vi "Msg Action.vi"(0 "TCP Server in":refnum<class "TCP Server.lvclass">, 1 "TCP Client ID":refnum<k5>, 2 "Sender IP":string, 5 "TCP Server Msg Actions":T1, 7 "uService ID":string, 9 "uService Class Name":string, 11 "error in (no error)":errorcluster) -> (4 "TCP Server out":refnum<class "TCP Server.lvclass">, 6 "External Error out":errorcluster, 15 "error out":errorcluster)   [LabVIEW 2026, in "TALOS.lvlib" / "TCP Server.lvlib" / "TCP Server.lvclass"]
uses:
  TCP Server.lvclass
  TCP Server Msg Actions.ctl
  C:/LabVIEW Code/TALOS/builds/Actor Framework PPL/Actor Framework.lvlibp/1abvi3w/vi.lib/ActorFramework/Actor/Actor.lvclass
  C:/LabVIEW Code/TALOS/talos/Father of all uServices/Father of all uServices/Father of all uServices.lvclass
  Ancestor/Ancestor/Ancestor.lvclass/Ancestor.ctl
  Guardian/Guardian Messages/Launch uService Msg/Launch uService Msg.lvclass/Launch uService Msg.ctl
  Guardian/Guardian Messages/Message to uService Msg/Message to uService Msg.lvclass/Message to uService Msg.ctl
  Guardian/Guardian Messages/TCP-SV Message Interpreter Msg/TCP-SV Message Interpreter Msg.lvclass/TCP-SV Message Interpreter Msg.ctl
  <vilib>/AdvancedString/Delimited String to 1D String Array (string).vi
  <vilib>/Utility/error.llb/Trim Whitespace (string).vi
  FGV/Error Memory/Get Error Description.vi
  Ancestor/Ancestor/Read ID.vi
  Support VIs/Get Class Name.vi
  Guardian/Guardian Messages/Message to uService Msg/Send Message to uService.vi
  <vilib>/Utility/error.llb/Trim Whitespace One-Sided.vi
  FGV/Error Memory/Error Memory Core.vi
  Support VIs/Circus Root Path.vi
  FGV/Error Memory/Error Crt Lvl checker.vi
  FGV/Error Memory/Error Memory Core.vi/40c8088d-b597-4017-91af-faa98e00292e.vi
  FGV/Error Memory/Error Memory Core.vi/d4a3ab98-063c-4e44-b43d-fbdcfe6c2be2.vi
  Father of all uServices/Father of all uServices/Father of all uServices.lvclass
  Support VIs/Global Memory.vi
  <vilib>/Utility/LVClass/Get LV Class Name.vi
  Support VIs/Is in Packed Library.vi
  Support VIs/TALOS Root path.vi
  Support VIs/Read CSV worksheet.vi
  Support VIs/Global Constants.vi
  <vilib>/Utility/error.llb/General Error Handler.vi
  Support VIs/Error Log.vi
  <vilib>/Utility/config.llb/Open Config Data.vi
  <vilib>/Utility/config.llb/Get Section Names.vi
  <vilib>/Utility/config.llb/Get Key Names.vi
  <vilib>/Utility/config.llb/Read Key.vi
  <vilib>/Utility/config.llb/Read Key (String).vi
  <vilib>/Utility/config.llb/Close Config Data.vi
  builds/Actor Framework PPL/Actor Framework.lvlibp/1abvi3w/vi.lib/ActorFramework/Message Enqueuer/Enqueue.vi
  Ancestor/Ancestor/Ancestor.lvclass
  <vilib>/Comparison/Equal/Equal Functor/Equal Functor.lvclass
  Guardian/Guardian Messages/Launch uService Msg/Launch uService Msg.lvclass
  Guardian/Guardian Messages/Message to uService Msg/Message to uService Msg.lvclass
  Guardian/Guardian Messages/TCP-SV Message Interpreter Msg/TCP-SV Message Interpreter Msg.lvclass
  builds/Actor Framework PPL/Actor Framework.lvlibp/1abvi3w/vi.lib/ActorFramework/Actor/Actor.lvclass
  TALOS.lvlib
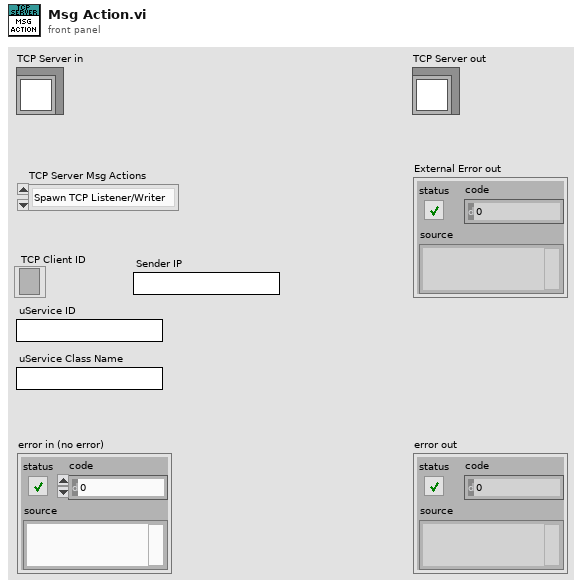
[diagram p1: front panel]
types:
  T1 = typedef "TALOS.lvlib/TCP Server.lvlib/TCP Server.lvclass/TCP Server Msg Actions.ctl" = enum16{"Spawn TCP Listener/Writer", "External Error", "I Exist", "Who the hell is this guy?", "Do nothing", "Are you the Bearer", "Farewell", "External Message"}
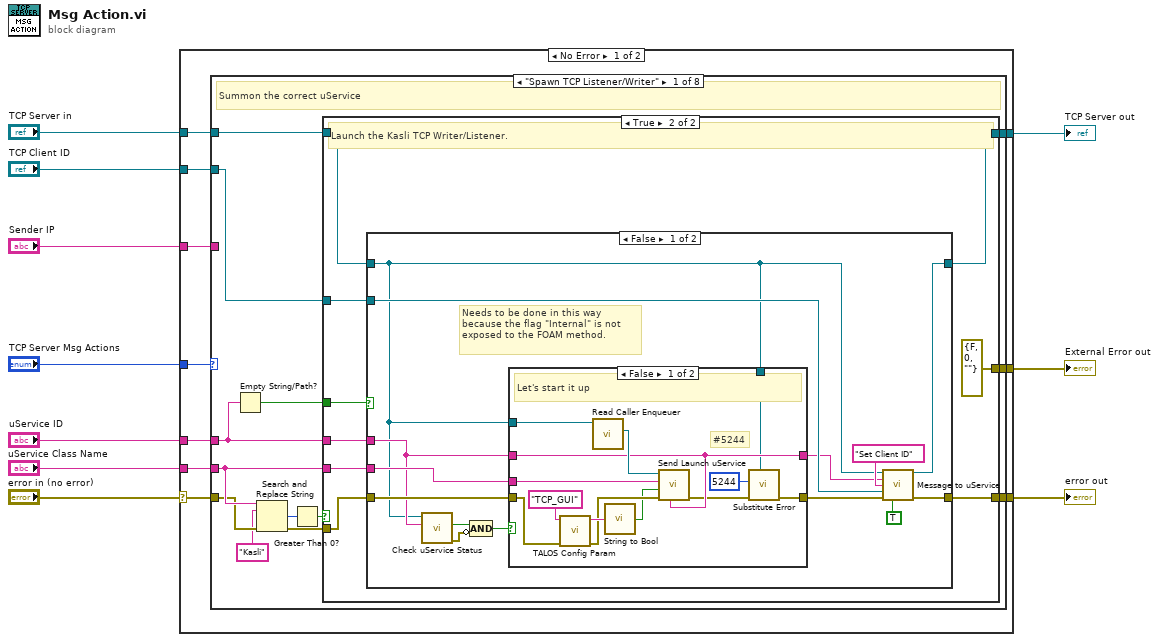
[diagram p0: block diagram]
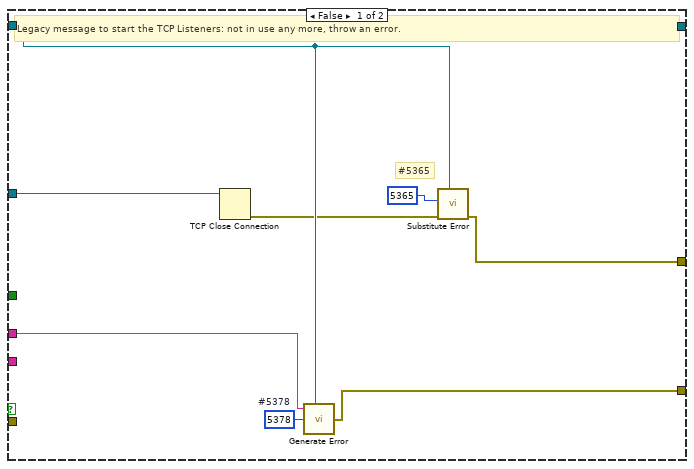
[diagram p2: hidden frame]
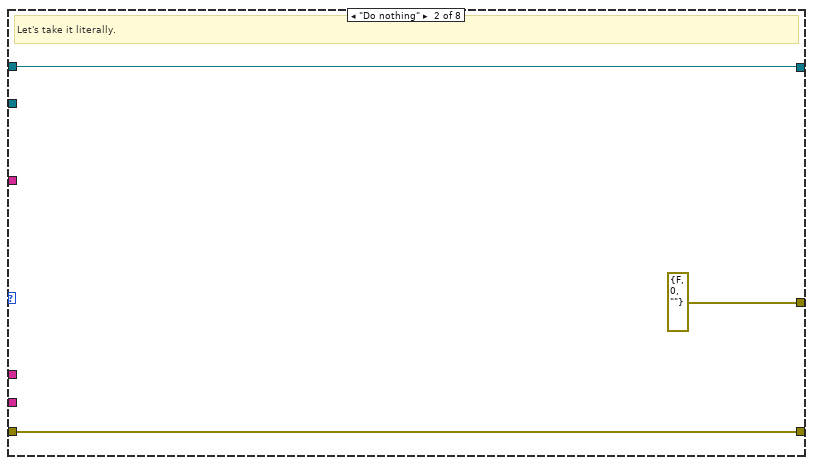
[diagram p5: hidden frame]
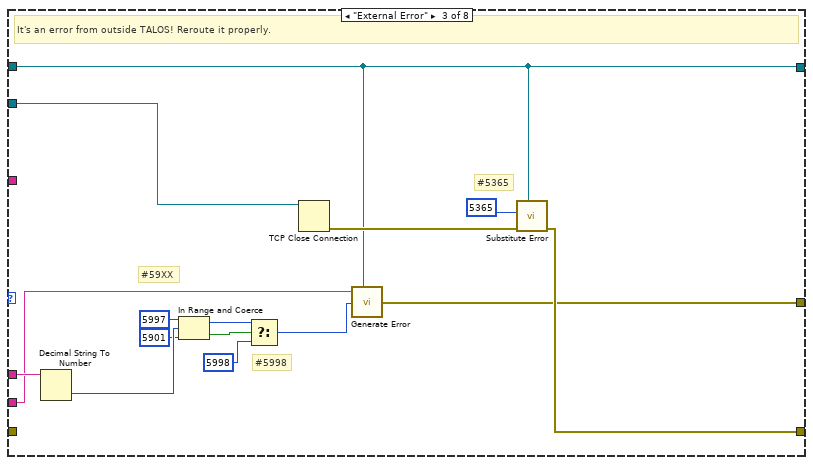
[diagram p6: hidden frame]
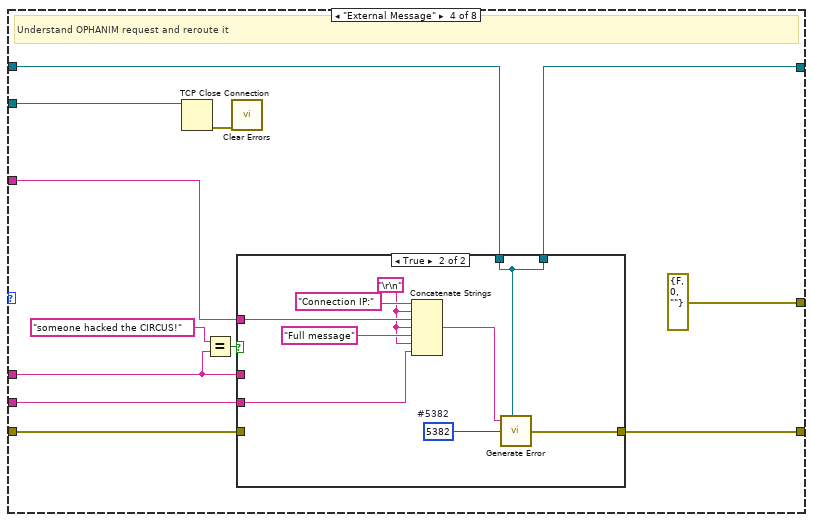
[diagram p7: hidden frame]
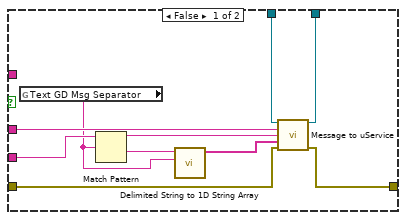
[diagram p8: hidden frame]
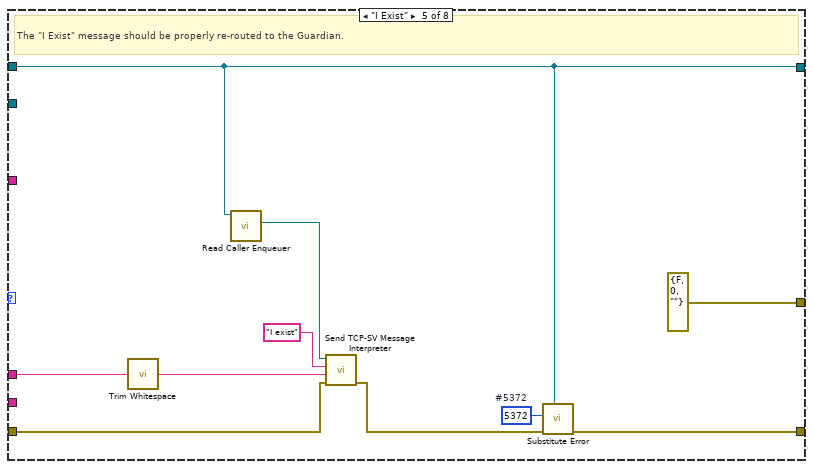
[diagram p9: hidden frame]
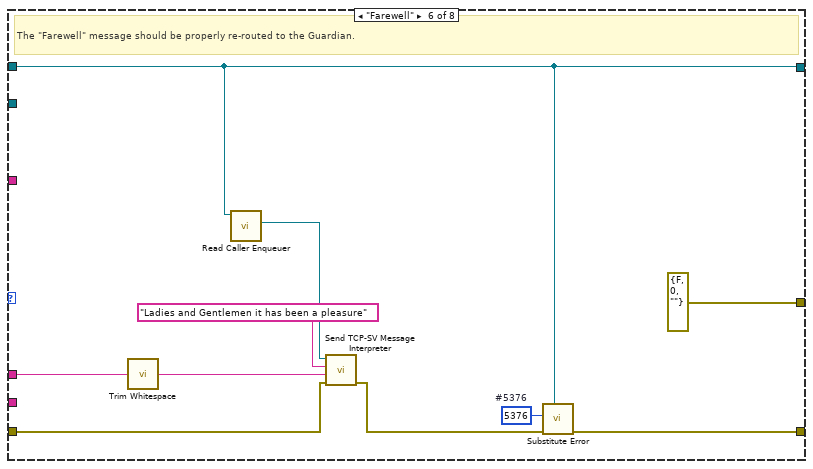
[diagram p10: hidden frame]
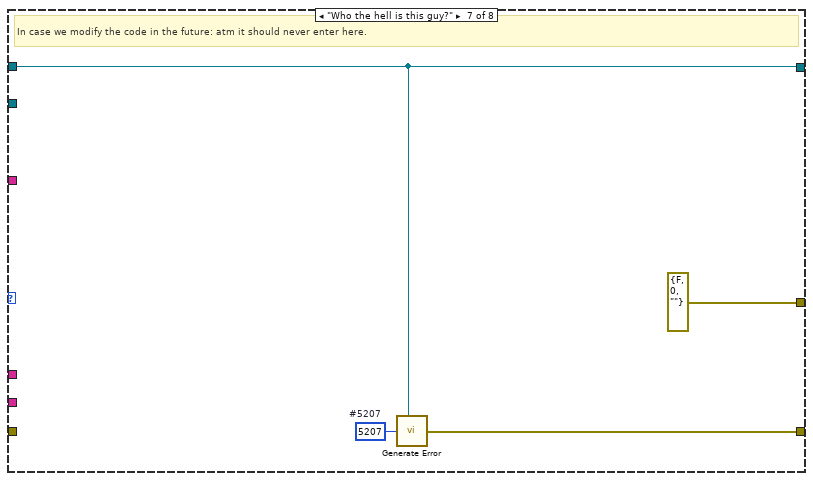
[diagram p11: hidden frame]
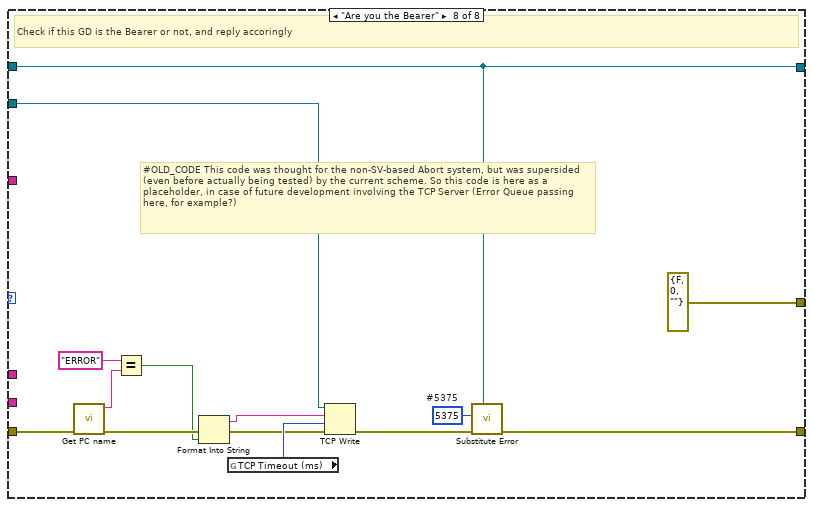
[diagram p12: hidden frame]
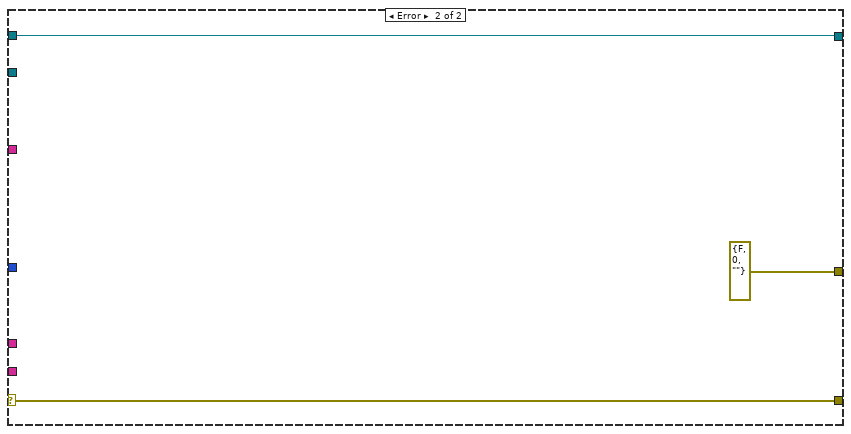
[diagram p13: hidden frame]
diagram:
  n1 = case shown="No Error" "error in (no error)" {
    selector: "error in (no error)" -> [w15 w170]
    tunnel: [w20 errorcluster {"status"=FALSE, "code"=0, "source"=""} ("error out")] -> w10
    tunnel: "TCP Server Msg Actions" -> [w19 _]
    tunnel: [w18 w171] -> w8
    tunnel: "uService Class Name" -> [w17 _]
    tunnel: "uService ID" -> [w16 _]
    tunnel: "TCP Server in" -> [w14 w171]
    tunnel: [w13 w170] -> w3
    tunnel: "TCP Client ID" -> [w12 _]
    tunnel: "Sender IP" -> [w11 _]
    frame No Error {
      n2 = case shown="\"Spawn TCP Listener/Writer\"" w19 {
        tunnel: w12 -> [w28 _ w99 w111 _ _ _ w167]
        tunnel: [w32 w83 w95 w104 w135 w145 w153 w163] -> w13
        tunnel: w14 -> [w29 w84 w94 w107 w133 w143 w151 w162]
        tunnel: w15 -> [w23 w83 _ w105 w136 w146 _ w160]
        tunnel: w16 -> [w33 _ w98 w101 w138 w148 _ _]
        tunnel: w17 -> [w27 _ w97 w106 _ _ _ _]
        tunnel: [w31 w84 w94 w108 w133 w143 w151 w162] -> w18
        tunnel: [w30 errorcluster {"status"=FALSE, "code"=0, "source"=""} ("error out") w85 errorcluster {"status"=FALSE, "code"=0, "source"=""} ("error out") errorcluster {"status"=FALSE, "code"=0, "source"=""} ("error out") errorcluster {"status"=FALSE, "code"=0, "source"=""} ("error out") errorcluster {"status"=FALSE, "code"=0, "source"=""} ("error out") errorcluster {"status"=FALSE, "code"=0, "source"=""} ("error out")] -> w20
        tunnel: w11 -> [_ _ _ w100 _ _ _ _]
        frame "Spawn TCP Listener/Writer" {
          # "Summon the correct uService"
          n3 = Empty String/Path?(string/path=w33) -> (empty?=w26:bool)
          n4 = Search and Replace String(input string=w27, search string="Kasli", error in=w23) -> (number of replacements=w25:i32, error out=w24:errorcluster)  [unwired: 5 in, 2 out]
          n5 = Greater Than 0?(x=w25) -> (x > 0?=w21:bool)
          n6 = case shown="True" w21 {
            tunnel: w28 -> [w37 w49]
            tunnel: [w41 w45] -> w32
            tunnel: w29 -> [w40 w50]
            tunnel: w33 -> [w35 w48]
            tunnel: [w40 w47] -> w31
            tunnel: [w39 errorcluster {"status"=FALSE, "code"=0, "source"=""} ("error out")] -> w30
            tunnel: w26 -> [_ w43]
            tunnel: w27 -> [_ w44]
            tunnel: w24 -> [_ w42]
            frame False {
              w34 = 5378  # #5378
              # "#5365"
              # "Legacy message to start the TCP Listeners: not in use any more, throw an error."
              n7 = TCP Close Connection(connection ID=w37) -> (error out=w38:errorcluster)  [unwired: 2 in, 1 out]
              n8 = call "Generate Error.vi"("Optional String"=w35, "Class"=w40, "Error Code"=w34) -> ("error out"=w41:errorcluster)  [unwired: 4 in]
              n9 = call "Substitute Error.vi"("LabVIEW Object"=w40, "error in (no error)"=w38, "Error Code"=5365) -> ("error out"=w39:errorcluster)  [unwired: 8 in]
            }
            frame True {
              # "Launch the Kasli TCP Writer/Listener."
              n10 = case shown="False" w43 {
                tunnel: w50 -> [w51 w80]
                tunnel: w42 -> [w62 w81]
                tunnel: w44 -> [w61 _]
                tunnel: w48 -> [w52 _]
                tunnel: w49 -> [w59 _]
                tunnel: [w57 w81] -> w45
                tunnel: [w54 w80] -> w47
                frame False {
                  # "Needs to be done in this way because the flag \"Internal\" is not exposed to the FOAM method."
                  n11 = call-dynamic "Check uService Status.vi"("uService ID"=w52, "Father of all uServices in"=w51) -> ("error out"=w64:errorcluster, "Online?"=w53:bool)  [unwired: 6 in, 2 out]
                  n12 = Compound Arithmetic op=AND(w53, invert w64) -> (w63:bool)
                  n13 = case shown="False" w63 {
                    tunnel: [w71 w79] -> w60
                    tunnel: w51 -> [w77 _]
                    tunnel: w62 -> [w67 w79]
                    tunnel: w52 -> [w74 w78]
                    tunnel: w61 -> [w75 _]
                    tunnel: [w74 w78] -> w56
                    tunnel: w51 -> [w70 _]
                    frame False {
                      # "#5244"
                      # "Let's start it up"
                      n14 = call "TALOS Config Param.vi"("error in (no error)"=w67, "Parameter Name"="TCP_GUI") -> ("error out"=w66:errorcluster, "Output"=w69:string)  [unwired: 8 in]
                      n15 = call "Read Caller Enqueuer.vi"("Actor"=w77) -> ("Caller Enqueuer"=w76:refnum<class "Message Enqueuer.lvclass">)  [unwired: 10 in]
                      n16 = call "String to Bool.vi"("String"=w69) -> ("Boolean"=w65:bool)
                      n17 = call "Send Launch uService.vi"("uService ID"=w74, "error in (no error)"=w66, "GUI?"=w65, "uService Class Name"=w75, "Message Enqueuer"=w76) -> ("error out"=w72:errorcluster)  [unwired: 5 in, 1 out]
                      n18 = call "Substitute Error.vi"("LabVIEW Object"=w70, "error in (no error)"=w72, "Error Code"=5244) -> ("error out"=w71:errorcluster)  [unwired: 8 in]
                    }
                    frame True {
                      # "It's present!"
                    }
                  }
                  n19 = call "Message to uService.vi"("Father of all uServices in"=w51, "uService ID"=w56, "Message"="Set Client ID" ("Item Name"), "Data"=w59, "error in (no error)"=w60, "Locale?"=TRUE) -> ("Father of all uServices out"=w54:refnum<class "TCP Server.lvclass">, "error out"=w57:errorcluster)  [unwired: 8 in]
                }
                frame True {
                  # "We are in locale, or an error occurred, so do nothing!"
                }
              }
            }
          }
        }
        frame "Do nothing" {
          # "Let's take it literally."
        }
        frame "External Error" {
          # "#5998"
          # "#59XX"
          # "#5365"
          # "It's an error from outside TALOS! Reroute it properly."
          n20 = Decimal String To Number(string=w98) -> (number=w92:i32)  [unwired: 2 in, 1 out]
          n21 = In Range and Coerce(upper limit=5997, x=w92, lower limit=5901) -> (coerced(x)=w88:i32, In Range?=w89:bool)
          n22 = Select(t=w88, s=w89, f=5998) -> (s? t:f=w87:i32)
          n23 = TCP Close Connection(connection ID=w99) -> (error out=w96:errorcluster)  [unwired: 2 in, 1 out]
          n24 = call "Generate Error.vi"("Optional String"=w97, "Class"=w94, "Error Code"=w87) -> ("error out"=w85:errorcluster)  [unwired: 4 in]
          n25 = call "Substitute Error.vi"("LabVIEW Object"=w94, "error in (no error)"=w96, "Error Code"=5365) -> ("error out"=w95:errorcluster)  [unwired: 8 in]
        }
        frame "External Message" {
          # "Understand OPHANIM request and reroute it"
          n26 = TCP Close Connection(connection ID=w111) -> (error out=w109:errorcluster)  [unwired: 2 in, 1 out]
          n27 = Equal?(x="someone hacked the CIRCUS!", y=w101) -> (x = y?=w103:bool)
          n28 = call <vilib>:"Clear Errors.vi"("error in (no error)"=w109) -> ()  [unwired: 5 in, 2 out]
          n29 = case shown="True" w103 {
            tunnel: w101 -> [w121 _]
            tunnel: [w120 w130] -> w108
            tunnel: w107 -> [w119 w130]
            tunnel: w106 -> [w118 w124]
            tunnel: w105 -> [w116 _]
            tunnel: [w115 w129] -> w104
            tunnel: w100 -> [_ w127]
            frame False {
              n30 = global read "Global Constants.vi" "Text GD Msg Separator"() -> (w112:string)
              n31 = Match Pattern(string=w118, regular expression=w112) -> (before substring=w117:string, after substring=w113:string)  [unwired: 1 in, 2 out]
              n32 = call-poly <vilib>:"Delimited String to 1D String Array.vi"("delimiter"=w112, "delimited string"=w113) -> ("string array"=w114:string[])  [unwired: 9 in]
              n33 = call "Message to uService.vi"("Father of all uServices in"=w119, "uService ID"=w121, "Message"=w117, "Data"=w114, "error in (no error)"=w116) -> ("Father of all uServices out"=w120:refnum<class "TCP Server.lvclass">, "error out"=w115:errorcluster)  [unwired: 9 in]
            }
            frame True {
              w122 = 5382  # #5382
              w125 = "\r\n"
              n34 = Concatenate Strings("Connection IP:" ("string"), w125, w127, w125, "Full message" ("string"), w125, w124) -> (w123:string)
              n35 = call "Generate Error.vi"("Optional String"=w123, "Class"=w130, "Error Code"=w122) -> ("error out"=w129:errorcluster)  [unwired: 4 in]
            }
          }
        }
        frame "I Exist" {
          w131 = 5372  # #5372
          # "The \"I Exist\" message should be properly re-routed to the Guardian."
          n36 = call-poly <vilib>:"Trim Whitespace.vi"("string"=w138) -> ("trimmed string"=w137:string)  [unwired: 1 in]
          n37 = call "Read Caller Enqueuer.vi"("Actor"=w133) -> ("Caller Enqueuer"=w140:refnum<class "Message Enqueuer.lvclass">)  [unwired: 10 in]
          n38 = call "Send TCP-SV Message Interpreter.vi"("error in (no error)"=w136, "Data"=w137, "Message"="I exist", "Message Enqueuer"=w140) -> ("error out"=w134:errorcluster)  [unwired: 6 in, 1 out]
          n39 = call "Substitute Error.vi"("LabVIEW Object"=w133, "error in (no error)"=w134, "Error Code"=w131) -> ("error out"=w135:errorcluster)  [unwired: 8 in]
        }
        frame "Farewell" {
          w141 = 5376  # #5376
          # "The \"Farewell\" message should be properly re-routed to the Guardian."
          n40 = call-poly <vilib>:"Trim Whitespace.vi"("string"=w148) -> ("trimmed string"=w147:string)  [unwired: 1 in]
          n41 = call "Read Caller Enqueuer.vi"("Actor"=w143) -> ("Caller Enqueuer"=w150:refnum<class "Message Enqueuer.lvclass">)  [unwired: 10 in]
          n42 = call "Send TCP-SV Message Interpreter.vi"("error in (no error)"=w146, "Data"=w147, "Message"="Ladies and Gentlemen it has been a pleasure", "Message Enqueuer"=w150) -> ("error out"=w144:errorcluster)  [unwired: 6 in, 1 out]
          n43 = call "Substitute Error.vi"("LabVIEW Object"=w143, "error in (no error)"=w144, "Error Code"=w141) -> ("error out"=w145:errorcluster)  [unwired: 8 in]
        }
        frame "Who the hell is this guy?" {
          w152 = 5207  # #5207
          # "In case we modify the code in the future: atm it should never enter here."
          n44 = call "Generate Error.vi"("Class"=w151, "Error Code"=w152) -> ("error out"=w153:errorcluster)  [unwired: 5 in]
        }
        frame "Are you the Bearer" {
          w165 = 5375  # #5375
          # "#OLD_CODE This code was thought for the non-SV-based Abort system, but was supersided (even before actually being tested) by the current scheme. So this code is here as a placeholder, in case of future development involving the TCP Server (Error Queue passing here, for example?)"
          # "Check if this GD is the Bearer or not, and reply accoringly"
          n45 = call "Get PC name.vi"("error in (no error)"=w160) -> ("error out"=w161:errorcluster, "Hostname"=w159:string)  [unwired: 9 in]
          n46 = Equal?(x="ERROR", y=w159) -> (x = y?=w157:bool)
          n47 = Format Into String(error in=w161, w157) -> (resulting string=w156:string, error out=w158:errorcluster)  [unwired: 2 in]
          n48 = global read "Global Constants.vi" "TCP Timeout (ms)"() -> (w168:i32)
          n49 = TCP Write(connection ID=w167, data in=w156, error in (no error)=w158, 9:w168) -> (error out=w164:errorcluster)  [unwired: 2 out]
          n50 = call "Substitute Error.vi"("LabVIEW Object"=w162, "error in (no error)"=w164, "Error Code"=w165) -> ("error out"=w163:errorcluster)  [unwired: 8 in]
        }
      }
    }
    frame Error {
    }
  }
  "External Error out" <- w10
  "TCP Server out" <- w8
  "error out" <- w3
